vi "ScrollATR.vi"(0 "reference in":refnum<vi>, 1 "Line to focus":string, 2 "error in":errorcluster) -> (3 "reference out":refnum<vi>, 4 "Line number":i32, 5 "OK?":bool, 6 "error out":errorcluster)   [LabVIEW 2017]
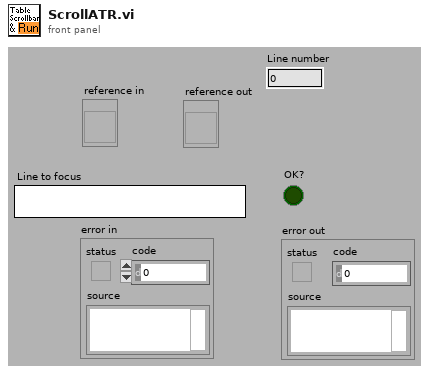
[diagram p1: front panel]
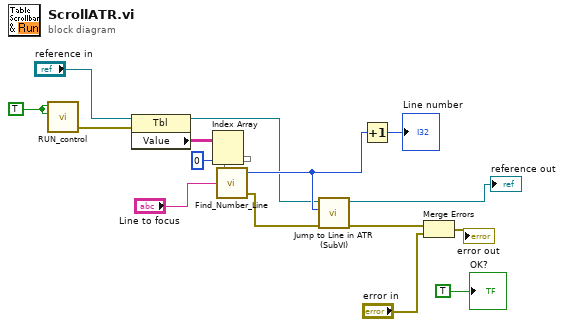
[diagram p0: block diagram]
diagram:
  w5 = TRUE ("Blinking")
  n1 = call "RUN_control.vi"("Blinking(:T)"=w5, "Value (:T)"=w5) -> ("error out"=w6:errorcluster)  [unwired: 3 in, 2 out]
  n2 = property on="Property Node" class="Tbl"(reference="reference in", error in=w6) -> (reference out=w7:refnum<vi>, "Value"=w3:string[][])  [unwired: 1 out]
  n3 = Index Array(array=w3, index (col)=0 ("disabled index (col)")) -> (element=w2:string[])  [unwired: 1 in]
  n4 = call "Find_Number_Line.vi"("Test Paragraph"="Line to focus", "Row Headers[]"=w2) -> ("error out"=w14:errorcluster, "Line number"=w16:i32)  [unwired: 1 in, 1 out]
  n5 = call "Jump to Line in ATR (SubVI).vi"("error in (no error)"=w14, "Line number"=w16, "Table in"=w7) -> ("error out"=w10:errorcluster, "Table out"=→"reference out":refnum<vi>)  [unwired: 7 in]
  n6 = Increment(x=w16) -> (x+1=→"Line number":i32)
  n7 = Merge Errors(w10, "error in") -> (→"error out":errorcluster)
  "OK?" <- TRUE ("OK?")
